vi "JudgeFullAngle1.vi"(6 "Auto":bool, 7 "Config":T1={"Difference"=0.005, "Repeate"=10.0, "PeakIndex"=0, "Name"=""} {"Repeate" format="%#_13g"; "Difference" format="%#_13g"}, 8 "Test Name":string(combo)="WDW", 9 "LastAngle":dbl, 10 "PlotName":i32(ring) items=["ForceDown"=0, "ForceUp"=6], 11 "XY Graph":cluster{"Angle Data":dbl[], "Array":dbl[]}[](array[cluster])) -> (0 "IndexOut":i32, 1 "AngleOut":dbl, 2 "ForceOut":dbl, 3 "Force Value":string)   [LabVIEW 2017]
panel:
  out "Counter":dbl
  out "ForceIndex":i32
  out "ForceMemory":dbl
  out "LengthScan":i32
  out "IndexStart":i32
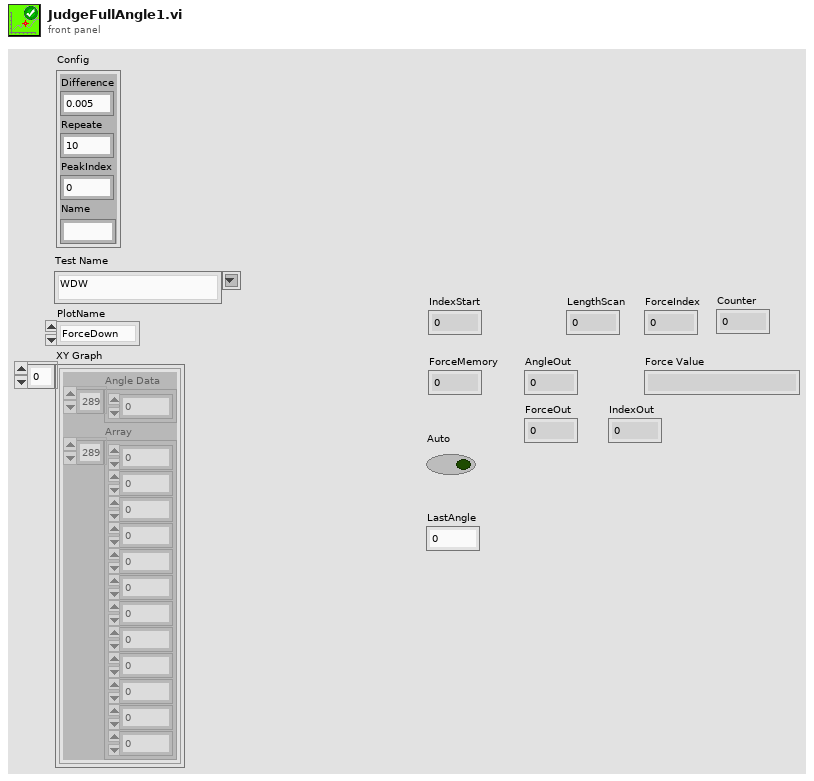
[diagram p1: front panel]
types:
  T1 = cluster{"Difference":dbl, "Repeate":dbl, "PeakIndex":i32, "Name":string}
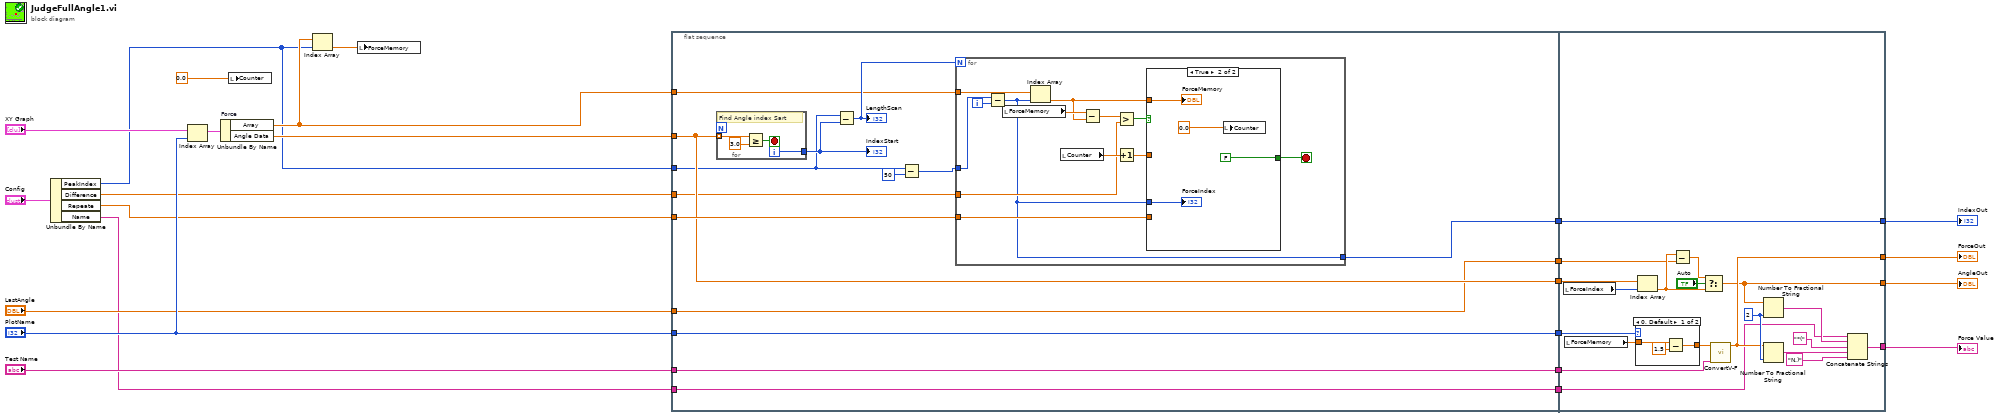
[diagram p0: block diagram]
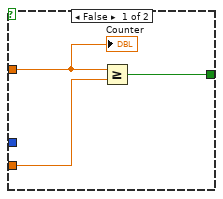
[diagram p2: hidden frame]
diagram:
  n1 = Unbundle By Name("Config") -> ("PeakIndex"=w8:i32, "Difference"=w12:dbl, "Repeate"=w11:dbl, "Name"=w2:string)
  n2 = Index Array(array="XY Graph", index="PlotName") -> (element=w24:cluster{"Angle Data":dbl[], "Array":dbl[]})
  n3 = Unbundle By Name "Force"(w24) -> ("Array"=w9:dbl[], "Angle Data"=w22:dbl[])
  n4 = local write "Counter"(0.0 ("ForceMemory")) -> ()
  n5 = Index Array(array=w9, index=w8) -> (element=w10:dbl)
  n6 = local write "ForceMemory"(w10) -> ()
  n7 = flat-sequence {
    tunnel: w22 -> [w34]
    tunnel: w9 -> [w37]
    tunnel: w11 -> [w35]
    tunnel: [w34] -> w7
    tunnel: "PlotName" -> [w33]
    tunnel: [w33] -> w6
    tunnel: "Test Name" -> [w32]
    tunnel: [w32] -> w5
    tunnel: w8 -> [w31]
    tunnel: w12 -> [w28]
    tunnel: [w27] -> w4
    tunnel: "LastAngle" -> [w26]
    tunnel: [w26] -> w3
    tunnel: w2 -> [w25]
    tunnel: [w25] -> w1
    tunnel: w7 -> [w82]
    tunnel: w6 -> [w80]
    tunnel: w5 -> [w77]
    tunnel: [w74] -> w18
    tunnel: [w76] -> w17
    tunnel: [w67] -> w16
    tunnel: w4 -> [w73]
    tunnel: [w73] -> w15
    tunnel: w3 -> [w64]
    tunnel: w1 -> [w63]
    frame #0 {
      n8 = for {
        tunnel: w34 -> [w62] mode=indexing
        tunnel: [w60] -> w36
        i -> [w60]
        stop <- w59 stop-if-true
        # "Find Angle index Sart"
        n9 = Greater Or Equal?(x=w62, y=3.0) -> (x >= y?=w59:bool)
      }
      "IndexStart" <- w36
      n10 = Subtract(x=w31, y=w36) -> (x-y=w38:i32)
      "LengthScan" <- w38
      n11 = Subtract(x=w31, y=50) -> (x-y=w30:i32)
      n12 = for {
        N: w38 -> [_]
        tunnel: w37 -> [w51]
        tunnel: w35 -> [w48]
        tunnel: w30 -> [w47]
        tunnel: w28 -> [w40]
        tunnel: [w39] -> w27
        i -> [w50]
        stop <- w49 stop-if-true
        n13 = Subtract(x=w47, y=w50) -> (x-y=w39:i32)
        n14 = local read "ForceMemory"() -> (w45:dbl)
        n15 = Index Array(array=w51, index=w39) -> (element=w44:dbl)
        n16 = local read "Counter"() -> (w42:dbl)
        n17 = Subtract(x=w45, y=w44) -> (x-y=w43:dbl)
        n18 = Greater?(x=w43, y=w40) -> (0:w46:bool)
        n19 = Increment(x=w42) -> (x+1=w41:dbl)
        n20 = case shown="True" w46 {
          tunnel: w44 -> [_ w58]
          tunnel: w39 -> [_ w57]
          tunnel: [w53 FALSE] -> w49
          tunnel: w48 -> [w54 _]
          tunnel: w41 -> [w52 _]
          frame False {
            n21 = Greater Or Equal?(x=w52, y=w54) -> (x >= y?=w53:bool)
            "Counter" <- w52
          }
          frame True {
            n22 = local write "Counter"(0.0 ("Counter")) -> ()
            "ForceMemory" <- w58
            "ForceIndex" <- w57
          }
        }
      }
    }
    frame #1 {
      w78 = i16 2 ("precision (6)")
      n23 = local read "ForceIndex"() -> (w81:i32)
      n24 = local read "ForceMemory"() -> (w79:dbl)
      n25 = case shown="0, Default" w80 {
        tunnel: [w84 w86] -> w75
        tunnel: w79 -> [w83 w86]
        frame 0, Default {
          n26 = Subtract(x=w83, y=1.5) -> (x-y=w84:dbl)
        }
        frame 6 {
        }
      }
      n27 = Index Array(array=w82, index=w81) -> (element=w65:dbl)
      n28 = Subtract(x=w65, y=w64) -> (x-y=w66:dbl)
      n29 = Select(t=w66, s="Auto", f=w65) -> (s? t:f=w67:dbl)
      n30 = call "ConvertV-F.vi"("Test Name"=w77, "Volt In"=w75) -> ("Force Out"=w74:dbl)  [unwired: 9 in]
      n31 = Number To Fractional String(number=w67, precision (6)=w78) -> (F-format string=w72:string)  [unwired: 2 in]
      n32 = Number To Fractional String(number=w74, precision (6)=w78) -> (F-format string=w70:string)  [unwired: 2 in]
      n33 = Concatenate Strings(w63, w72, "*(" ("string"), w70, "N.)" ("string")) -> (w76:string)
    }
  }
  "AngleOut" <- w16
  "Force Value" <- w17
  "ForceOut" <- w18
  "IndexOut" <- w15
